vi "Read ADC Datas.vi"(8 "error in (no error)":errorcluster, 9 "length":u32, 10 "buffer":string, 11 "channel":i8) -> (0 "error out":errorcluster, 2 "buffer out":string, 3 "function return":u32)   [LabVIEW 2021, in "vmmso.lvlib"]
doc: "DLL_API unsigned int WINAPI ReadADCDatas(char channel, unsigned char* buffer, unsigned int length);"
uses:
  vmmso.lvlib
  vmmso.dll
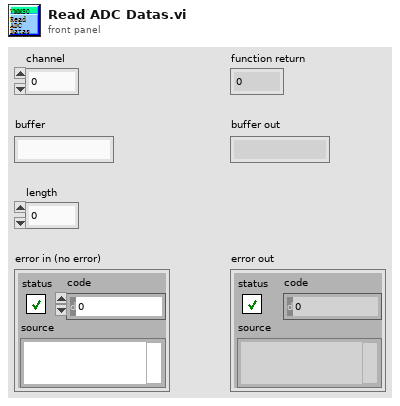
[diagram p1: front panel]
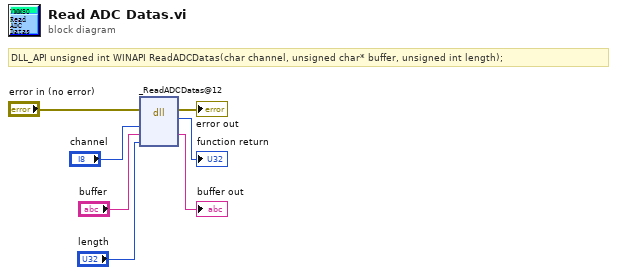
[diagram p0: block diagram]
diagram:
  # "DLL_API unsigned int WINAPI ReadADCDatas(char channel, unsigned char* buffer, unsigned int length);"
  n1 = dll-call lib="O:/MSO/library/demo-Labview/vmmso/vmmso.*" fn="_ReadADCDatas@12"(error in="error in (no error)", "channel"="channel", "buffer"="buffer", "length"="length") -> (error out=→"error out":errorcluster, →"function return":u32, "buffer"=→"buffer out":string)  [unwired: 4 in, 1 out]
